vi "DSF.Engine.Memory.Cache.Framework.Get Plugin Cache.vi"(10 "Plugin ID":i32, 11 "Framework Cache in":refnum<class "DSF.Engine.Memory.Cache.Framework.lvclass">) -> (2 "Plugin Cache":refnum<class "DSF.Engine.Memory.Cache.Plugin.lvclass">, 3 "Framework Cache out":refnum<class "DSF.Engine.Memory.Cache.Framework.lvclass">)   [LabVIEW 2016, in "DSF.Engine.lvlib" / "DSF.Engine.Memory.Cache.Framework.lvclass"]
uses:
  DSF.Engine.Memory.Cache.Framework.lvclass
  DSF.Engine.Memory.Cache.Plugin.lvclass
  DSF.Engine.Memory.Cache.Framework.lvclass/DSF.Engine.Memory.Cache.Framework.ctl
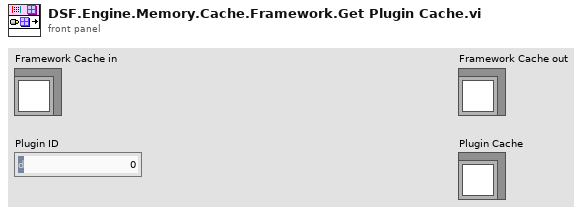
[diagram p1: front panel]
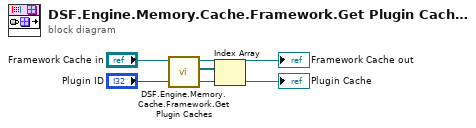
[diagram p0: block diagram]
diagram:
  n1 = call "DSF.Engine.Memory.Cache.Framework.Get Plugin Caches.vi"("Framework Cache in"="Framework Cache in") -> ("Plugin Caches"=w1:refnum<class "DSF.Engine.Memory.Cache.Plugin.lvclass">[], "Framework Cache out"=→"Framework Cache out":refnum<class "DSF.Engine.Memory.Cache.Framework.lvclass">)  [unwired: 9 in]
  n2 = Index Array(array=w1, index="Plugin ID") -> (element=→"Plugin Cache":refnum<class "DSF.Engine.Memory.Cache.Plugin.lvclass">)
